vi "BotSpeak_RIO_PBtns.vi"(4 "Bot Settings":T1) -> (0 "Btns":T2, 1 "Bot Settings 2":T1)   [LabVIEW 2012]
doc: "Retrieves the state of each of the RIO's 5 buttons and returns a cluster of 5 booleans corresponding to the state of each button."
uses:
  <userlib>/BotSpeak/VIs/Direct/BotSpeak_Control.ctl
panel:
  out "response":string="169.254.32.85"
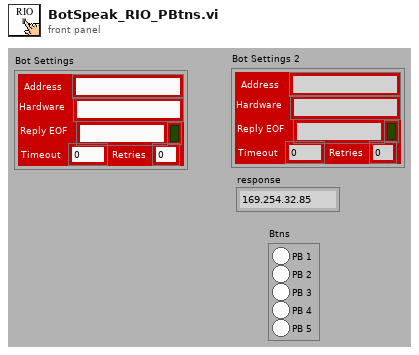
[diagram p1: front panel]
types:
  T1 = typedef "BotSpeak_Control.ctl" = cluster{"Address":string, "Reply EOF":string, "Hardware":string, "Retries":i8, "Timeout":i32, "Open?":bool}
  T2 = cluster{"PB 1":bool, "PB 2":bool, "PB 3":bool, "PB 4":bool, "PB 5":bool}
  T3 = cluster{"Boolean array[0]":bool, "Boolean array[1]":bool, "Boolean array[2]":bool, "Boolean array[3]":bool, "Boolean array[4]":bool}
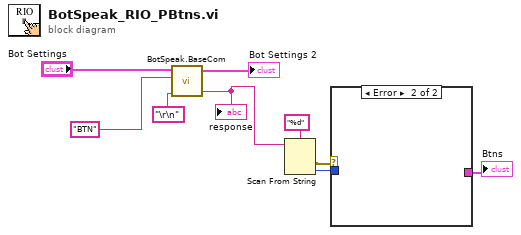
[diagram p0: block diagram]
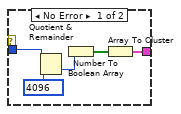
[diagram p2: hidden frame]
diagram:
  n1 = call <userlib>:"BotSpeak.BaseCom.vi"("Termination"="\r\n", "command"="BTN", "Bot Settings in"="Bot Settings") -> ("response"=w2:string, "Bot Settings out"=→"Bot Settings 2":T1)  [unwired: 2 in]
  "response" <- w2
  n2 = Scan From String(format string="%d", input string=w2) -> (error out=w6:errorcluster, output 1=w8:i32)  [unwired: 3 in, 2 out]
  n3 = case shown="Error" w6 {
    tunnel: w8 -> [w12 _]
    tunnel: [w13 _] -> w7
    frame No Error {
      n4 = Quotient & Remainder(x=w12, y=4096) -> (floor(x/y)=w11:i32)  [unwired: 1 out]
      n5 = Number To Boolean Array(number=w11) -> (Boolean array=w14:bool[])
      n6 = Array To Cluster(array=w14) -> (cluster=w13:T3)
    }
    frame Error {
    }
  }
  "Btns" <- w7
